vi "Espinoza_Lab_5.vi"() -> ()   [LabVIEW 2010]
uses:
  <vilib>/Utility/file.llb/Write To Spreadsheet File (I64).vi
panel:
  out "Peak to Peak":u16
  in  "Board Number":i32
  in  "Auto Save Data":bool=TRUE
  out "Date/Time String":string="2012-02-20 12-35.08"
  in  "Time Format String (%c)":string="%Y-%m-%d %H-%M.%S"
  in  "Data File Path Ending":string=".dat"
  out "Previous Acquistion":u16[](graph)
  out "ErrMsg":string="No error has occurred"
  out "ErrCode":i32
  out "Current Acquisition":u16[](graph)
  in  "InterChannel Delay":sgl=-1.0 format="%.2f"
  in  "Range":i32(ring)=1 items=["Not Programmable"=0, "+- 20 V"=27, "+- 10 V"=1, "+- 5 V"=2, "+- 4 V"=28, "+- 2.5 V"=3, "+- 2 V"=29, "+- 1.67 V"=4, "+- 1.25 V"=5, "+- 1 V"=6, "+- .625 V"=7, "+- .5 V"=8, "+- .25 V"=30, "+- .2 V"=31, "+- .1 V"=9, "+- .05 V"=10, "+- .01 V"=11, "+- .005 V"=12, "0 - 10 V"=13, "0 - 5 V"=14, "0 - 4 V"=36, "0 - 2.5 V"=15, "0 - 2 V"=16, "0 - 1.67 V"=17, "0 - 1.25 V"=18, "0 - 1 V"=19, "0 - .5 V"=32, "0 - .25 V"=33, "0 - .2 V"=34, "0 - .1 V"=20, "0 - .02 V"=35, "0 - .01 V"=21, "4 - 20 mA"=22, "2 - 10 mA"=23, "1 - 5 mA"=24, ".5 - 2.5 mA"=25, "0 - 20 mA"=26]
  in  "Options":i32
  in  "Rate":i32
  in  "Count":i32
  in  "LowChan":i32
  in  "HighChan":i32
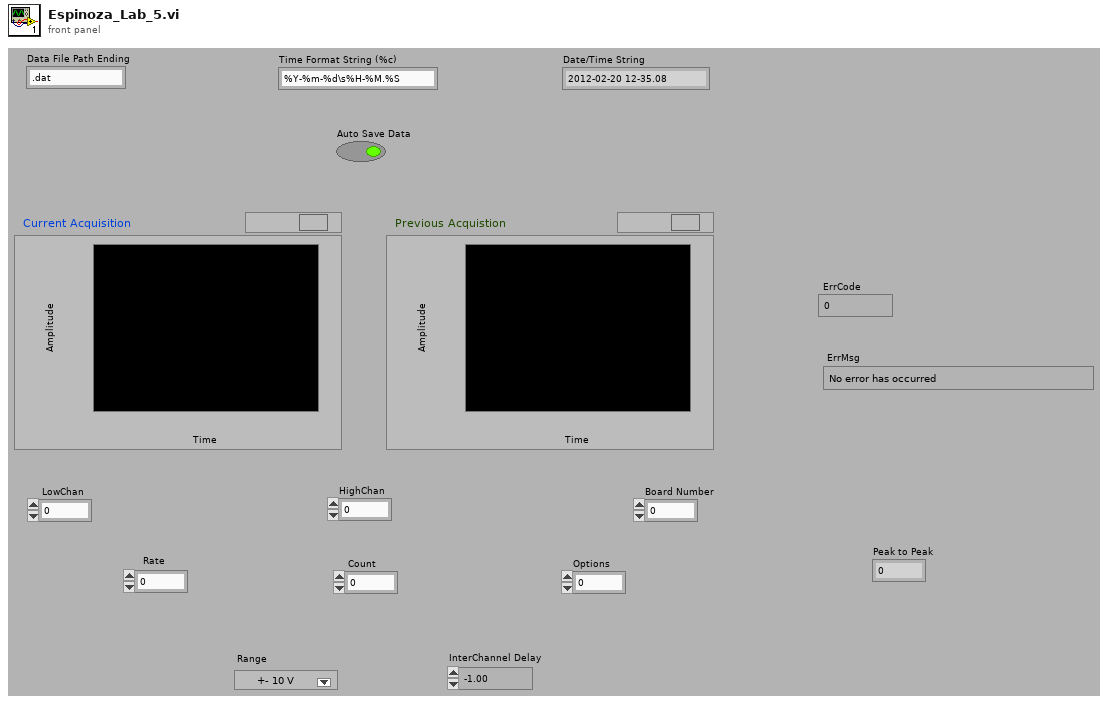
[diagram p1: front panel]
types:
  T1 = typedef "imagedata.ctl" = cluster{"image type":i32, "image depth":i32, "image":u8[], "mask":u8[], "colors":u32[], "Rectangle":cluster{"left":i16, "top":i16, "right":i16, "bottom":i16}}
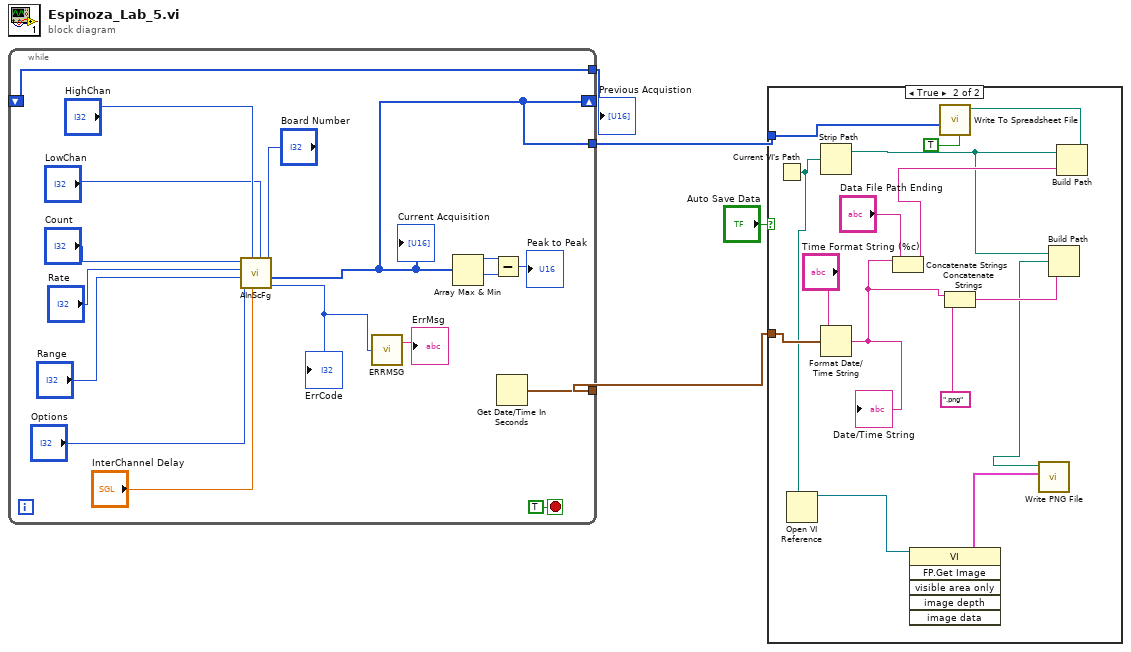
[diagram p0: block diagram]
diagram:
  n1 = while {
    shift-right: [w8] -> _
    shift-left: _ -> [w11]
    tunnel: [w11] -> w4
    tunnel: [w8] -> w1
    tunnel: [w10] -> w2
    stop <- TRUE stop-if-true
    n2 = call <menus>:"AInScFg.VI"("BoardNum"="Board Number", "LowChan"="LowChan", "InterChannel Delay"="InterChannel Delay", "HighChan"="HighChan", "Options"="Options", "Range"="Range", "Rate"="Rate", "Count"="Count") -> ("ErrCode"=w12:i32, "ADData"=w8:u16[])  [unwired: 1 out]
    "Current Acquisition" <- w8
    "ErrCode" <- w12
    n3 = call <menus>:"ERRMSG.VI"("ErrCode"=w12) -> ("ErrMsg"=→"ErrMsg":string)  [unwired: 1 out]
    n4 = Array Max & Min(array=w8) -> (max value=w6:u16, min value=w7:u16)  [unwired: 2 out]
    n5 = Subtract(x=w6, y=w7) -> (x-y=→"Peak to Peak":u16)
    n6 = Get Date/Time In Seconds() -> (seconds since 1Jan1904=w10:timestamp)
  }
  "Previous Acquistion" <- w4
  n7 = case shown="True" "Auto Save Data" {
    tunnel: w1 -> [_ w36]
    tunnel: w2 -> [_ w35]
    frame False {
    }
    frame True {
      n8 = Current VI's Path() -> (path=w27:path)
      n9 = Open VI Reference(vi path=w27) -> (vi reference=w28:refnum<vi>)  [unwired: 5 in, 1 out]
      n10 = Strip Path(path=w27) -> (stripped path=w26:path)  [unwired: 1 out]
      n11 = Format Date/Time String(time format string (%c)="Time Format String (%c)", seconds (now)=w35) -> (date/time string=w25:string)  [unwired: 1 in]
      "Date/Time String" <- w25
      n12 = Concatenate Strings(w25, "Data File Path Ending") -> (w32:string)
      n13 = invoke class="VI" method="FP.Get Image"(reference=w28) -> ("image data"=w29:T1)  [unwired: 5 in, 5 out]
      n14 = Concatenate Strings(w25, ".png" ("string")) -> (w23:string)
      n15 = Build Path(base path=w26, name or relative path=w23) -> (appended path=w22:path)
      n16 = call <vilib>:"Write PNG File.vi"("image data"=w29, "path to PNG file"=w22) -> ()  [unwired: 8 in, 2 out]
      n17 = Build Path(base path=w26, name or relative path=w32) -> (appended path=w31:path)
      n18 = call-poly <vilib>:"Write To Spreadsheet File.vi"("transpose? (no:F)"=TRUE, "1D data"=w36, "file path (dialog if empty)"=w31) -> ()  [unwired: 5 in, 1 out]
    }
  }
